vi "Wait4Flag(reentrant).vi"(8 "Raise Flag ?":bool, 11 "Ctl Refnum IN":refnum<vi>) -> (0 "Flag Value":bool, 3 "Ctl Refnum OUT":refnum<vi>)   [LabVIEW 2019]
panel:
  out "error out":errorcluster
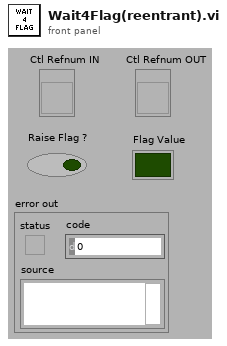
[diagram p1: front panel]
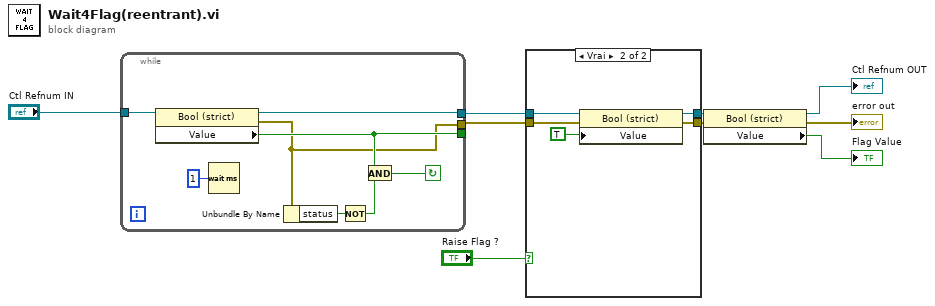
[diagram p0: block diagram]
diagram:
  n1 = while {
    tunnel: "Ctl Refnum IN" -> [w17]
    tunnel: [w11] -> _
    tunnel: [w13] -> w8
    tunnel: [w10] -> w7
    stop <- w15 continue-if-true
    n2 = property on="Property Node" class="Bool (strict)"(reference=w17) -> (reference out=w13:refnum<vi>, error out=w10:errorcluster, "Value"=w11:bool)  [unwired: 1 in]
    n3 = Wait (ms)(milliseconds to wait=u32 1) -> ()  [unwired: 1 out]
    n4 = Unbundle By Name(w10) -> ("status"=w16:bool)
    n5 = Not(x=w16) -> (.not. x?=w14:bool)
    n6 = And(x=w11, y=w14) -> (x .and. y?=w15:bool)
  }
  n7 = case shown="Vrai" "Raise Flag ?" {
    tunnel: w8 -> [w19 w24]
    tunnel: w7 -> [w18 w23]
    tunnel: [w19 w22] -> w5
    tunnel: [w18 w21] -> w4
    frame False {
    }
    frame True {
      n8 = property on="Property Node" class="Bool (strict)"(reference=w24, error in=w23, "Value"=TRUE) -> (reference out=w22:refnum<vi>, error out=w21:errorcluster)
    }
  }
  n9 = property on="Property Node" class="Bool (strict)"(reference=w5, error in=w4) -> (reference out=→"Ctl Refnum OUT":refnum<vi>, error out=→"error out":errorcluster, "Value"=→"Flag Value":bool)
